vi "Begin.vi"() -> (0 "error out":errorcluster)   [LabVIEW 2011]
doc: "Called before other user functions, this VI is expected to open initial I/O refnums, load in file data, and do all program initialization. Notice that the <B>error out</B> terminal is simply used for data flow. Wiring it to other structures or subVIs ensures that this VI runs first."
uses:
  <vilib>/Rock Robotics/WPI/Camera/WPI_CameraImageSize.ctl
  <vilib>/Rock Robotics/WPI/MotorControl/WPI_MotorControlDeviceRef.ctl
  <vilib>/Rock Robotics/SystemInterfaces/Typedef/FPGA_TypedefDigitalModule.ctl
  <vilib>/Rock Robotics/SystemInterfaces/DIO/FPGA_DIOPWMChannel.ctl
  <vilib>/Rock Robotics/WPI/PWM/WPI_PWMDeadband.ctl
  <vilib>/Rock Robotics/WPI/CAN/Jaguar/SubVIs/WPI_CANJaguar_ControlMode.ctl
  <vilib>/Rock Robotics/WPI/PWM/WPI_PWMTransform_ConPane.ctl
  PIDCluster.ctl
  <vilib>/Rock Robotics/SystemInterfaces/DIO/FPGA_DIORelayChannel.ctl
  <vilib>/Rock Robotics/WPI/Solenoid/WPI_SolenoidChannel.ctl
  <vilib>/Rock Robotics/SystemInterfaces/DIO/FPGA_DIOChannel.ctl
  <vilib>/Rock Robotics/WPI/Camera/WPI_CameraFrameRate.ctl
  <vilib>/Rock Robotics/WPI/Camera/WPI_CameraExposure Values.ctl
  <vilib>/Rock Robotics/WPI/Camera/WPI_CameraWhite Balance Values.ctl
  <vilib>/Rock Robotics/SystemInterfaces/AI/FPGA_AIGyroChannel.ctl
  <vilib>/Rock Robotics/SystemInterfaces/Typedef/FPGA_TypedefAnalogModule.ctl
  <vilib>/Rock Robotics/WPI/Joystick/WPI_JoystickDeviceEnum.ctl
  <vilib>/Rock Robotics/SystemInterfaces/Typedef/FPGA_TypedefSolenoidModule.ctl
  <vilib>/Rock Robotics/WPI/Solenoid/WPI_SolenoidOpenSingle.vi
  <vilib>/Rock Robotics/WPI/Counter/WPI_CounterDigitalInputToDigitalSource.vi
  <vilib>/Rock Robotics/WPI/Counter/WPI_CounterOpen UpDown Mode.vi
  <vilib>/Rock Robotics/WPI/MotorControl/WPI_MotorControlOpen Victor.vi
  <vilib>/Rock Robotics/WPI/MotorControl/WPI_MotorControlOpen Jaguar.vi
  <vilib>/Rock Robotics/WPI/Compressor/WPI_CompressorGetSetRefNum.vi
  <vilib>/Rock Robotics/WPI/Relay/WPI_RelayValue.ctl
  <vilib>/Rock Robotics/WPI/Relay/WPI_RelayDirection.ctl
panel:
  out "MotorControlDeviceRef":T1={"DeviceStatus"={"status"=FALSE, "code"=0, "source"=""}, "Type"=enum."PWM", "PWM"={"Digital Module"=enum."Digital Module 1", "PWM Channel"=enum."Invalid", "DeadBand"={"Name"="", "maxPositivePwm"=0, "minPositivePwm"=0, "centerPwm"=0, "maxNegativePwm"=0, "minNegativePwm"=0, "angularRange"=0}}, "CAN"={"Device Number"=0, "Control Mode"=enum."Percent VBus", "Semaphore"=refnum, "Max Vout"=12.0}, "Invert"=FALSE, "TransformRef"=refnum, "InvTransformRef"=refnum}
  in  "Image Size":T8=enum."320x240"
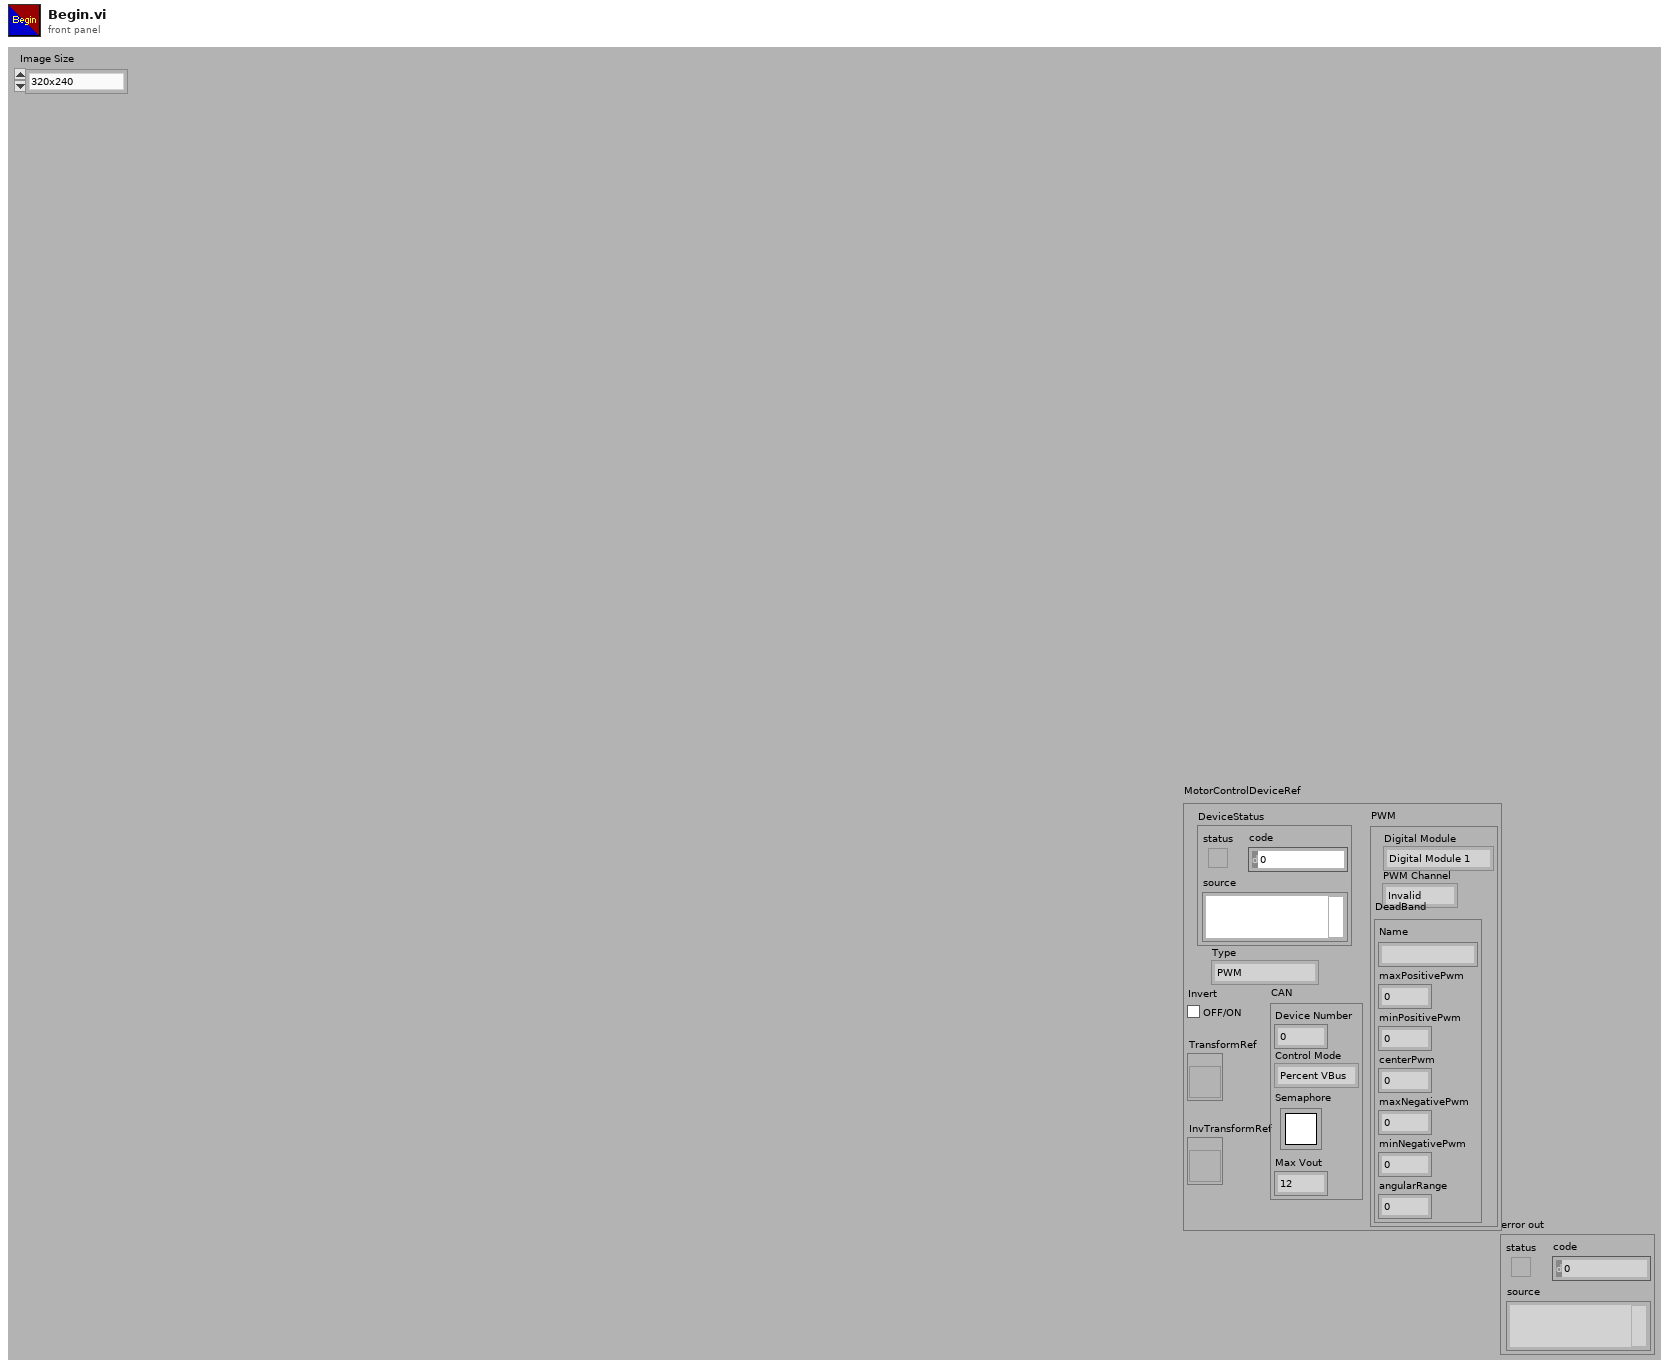
[diagram p1: front panel]
types:
  T1 = typedef "WPI_MotorControlDeviceRef.ctl" = cluster{"DeviceStatus":errorcluster, "Type":enum16{"PWM", "CAN"}, "PWM":cluster{"Digital Module":T2, "PWM Channel":T3, "DeadBand":T4}, "CAN":cluster{"Device Number":u8, "Control Mode":T5, "Semaphore":T6, "Max Vout":dbl}, "Invert":bool, "TransformRef":T7, "InvTransformRef":T7}
  T2 = typedef "FPGA_TypedefDigitalModule.ctl" = enum16{"Digital Module 1", "Digital Module 2"}
  T3 = typedef "FPGA_DIOPWMChannel.ctl" = enum8{"PWM 1", "PWM 2", "PWM 3", "PWM 4", "PWM 5", "PWM 6", "PWM 7", "PWM 8", "PWM 9", "PWM 10", "Invalid"}
  T4 = typedef "WPI_PWMDeadband.ctl" = cluster{"Name":string, "maxPositivePwm":i32, "minPositivePwm":i32, "centerPwm":i32, "maxNegativePwm":i32, "minNegativePwm":i32, "angularRange":u16}
  T5 = typedef "WPI_CANJaguar_ControlMode.ctl" = enum8{"Percent VBus", "Current", "Speed", "Position", "Voltage"}
  T6 = typedef "Semaphore RefNum" = refnum<k1>
  T7 = typedef "WPI_PWMTransform_ConPane.ctl" = refnum<vi>
  T8 = typedef "WPI_CameraImageSize.ctl" = enum16{"640x480", "320x240", "160x120"}
  T9 = typedef "PIDCluster.ctl" = cluster{"P":dbl, "I":dbl, "D":dbl}
  T10 = typedef "FPGA_DIORelayChannel.ctl" = enum8{"Relay 1", "Relay 2", "Relay 3", "Relay 4", "Relay 5", "Relay 6", "Relay 7", "Relay 8", "Invalid"}
  T11 = typedef "WPI_SolenoidChannel.ctl" = enum8{"Solenoid 1", "Solenoid 2", "Solenoid 3", "Solenoid 4", "Solenoid 5", "Solenoid 6", "Solenoid 7", "Solenoid 8", "Invalid"}
  T12 = typedef "FPGA_TypedefSolenoidModule.ctl" = enum16{"Solenoid Module 1", "Solenoid Module 2"}
  T13 = typedef "FPGA_DIOChannel.ctl" = enum8{"DIO 1", "DIO 2", "DIO 3", "DIO 4", "DIO 5", "DIO 6", "DIO 7", "DIO 8", "DIO 9", "DIO 10", "DIO 11", "DIO 12", "DIO 13", "DIO 14", "Invalid"}
  T14 = typedef "WPI_CameraFrameRate.ctl" = u32
  T15 = typedef "WPI_CameraExposure Values.ctl" = enum16{"Auto", "Flicker-free 50 Hz", "Flicker-free 60 Hz", "Hold current"}
  T16 = typedef "WPI_CameraWhite Balance Values.ctl" = enum16{"Auto", "Fixed indoor", "Fixed outdoor 1", "Fixed outdoor 2", "Fixed fluorescent 1", "Fixed fluorescent 2", "Hold current"}
  T17 = typedef "FPGA_AIGyroChannel.ctl" = enum8{"AI 1", "AI 2", "Invalid"}
  T18 = typedef "FPGA_TypedefAnalogModule.ctl" = enum16{"Analog Module 1", "Analog Module 2"}
  T19 = typedef "WPI_JoystickDeviceEnum.ctl" = enum16{"USB 1", "USB 2", "USB 3", "USB 4", "Kinect 1", "Kinect 2"}
  T20 = typedef "WPI_RelayDirection.ctl" = enum16{"Both directions", "Forward only", "Reverse only"}
  T21 = typedef "WPI_RelayValue.ctl" = enum16{"Off", "On", "Forward", "Reverse"}
  T22 = typedef "WPI_I2CDevRef.ctl" = cluster{"DevStatus":errorcluster, "Digital Module":T2, "Device Address":u8}
  T23 = typedef "WPI_DigitalInputDevRef.ctl" = cluster{"DevStatus":errorcluster, "DIO Channel":T13, "Digital Module":T2}
  T24 = typedef "FPGA_CounterEncoderSourceConvertionLVSourceType.ctl" = cluster{"DevStatus":errorcluster, "AnalogTriggerMode?":bool, "DigitalMode":cluster{"Digital Module":T2, "DIO Channel":T25}, "AnalogTriggerMode":cluster{"AnalogTriggerIndex":T26, "OutputType":T27}}
  T25 = typedef "FPGA_DIODigitalSourceChannel.ctl" = enum8{"DIO 1", "DIO 2", "DIO 3", "DIO 4", "DIO 5", "DIO 6", "DIO 7", "DIO 8", "DIO 9", "DIO 10", "DIO 11", "DIO 12", "DIO 13", "DIO 14", "Disabled"}
  T26 = typedef "FPGA_AnalogTriggerIndex.ctl" = enum8{"Trig 0", "Trig 1", "Trig 2", "Trig 3", "Trig 4", "Trig 5", "Trig 6", "Trig 7", "Invalid"}
  T27 = typedef "FPGA_AnalogTriggerOutType.ctl" = enum16{"InWindow", "TriggerState", "Rising", "Falling"}
  T28 = typedef "WPI_SolenoidDevRef.ctl" = cluster{"DevStatus":errorcluster, "Solenoid Module":T12, "Forward Solenoid Channel":T11, "Reverse Solenoid Channel":T11}
  T29 = typedef "WPI_CounterDevRef.ctl" = cluster{"DevStatus":errorcluster, "CntIndex":T30}
  T30 = typedef "FPGA_CounterCtrSystemIndex.ctl" = enum8{"Ctr 0", "Ctr 1", "Ctr 2", "Ctr 3", "Ctr 4", "Ctr 5", "Ctr 6", "Ctr 7", "Invalid"}
  T31 = typedef "WPI_GyroDevRef.ctl" = cluster{"DevStatus":errorcluster, "Analog Module":T18, "Analog Channel":T32, "Offset":dbl, "Gain (VoltsPerDegree/Second)":dbl}
  T32 = typedef "FPGA_AIChannel.ctl" = enum8{"AI 1", "AI 2", "AI 3", "AI 4", "AI 5", "AI 6", "AI 7", "AI 8", "Invalid"}
  T33 = typedef "WPI_CompressorDevRef.ctl" = cluster{"DevStatus":errorcluster, "DigitalInputDevRef":T23, "RelayDevRef":T34}
  T34 = typedef "WPI_RelayDevRef.ctl" = cluster{"DevStatus":errorcluster, "Relay Channel":T10, "Digital Module":T2, "Relay Direction":T20}
  T35 = typedef "WPI_DigitalOutputDevRef.ctl" = cluster{"Digital Module":T2, "DIO Channel":T13, "DevStatus":errorcluster}
  T36 = typedef "WPI_CameraDevRef.ctl" = cluster{"Camera Address":string, "CameraStatus":errorcluster, "Acquire Image Notifier":refnum<notifier>}
  T37 = typedef "WPI_JoystickDevRef.ctl" = cluster{"Device":T19}
  T38 = typedef "WPI_EncoderDevRef.ctl" = cluster{"DevStatus":errorcluster, "EncoderIndex":T39, "CounterIndex":T30, "DistancePerCount":dbl, "Decoding Type":T40}
  T39 = typedef "FPGA_EncoderIdx.ctl" = enum8{"Enc 0", "Enc 1", "Enc 2", "Enc 3", "Invalid"}
  T40 = typedef "WPI_EncoderType.ctl" = enum16{"1x", "2x", "4x"}
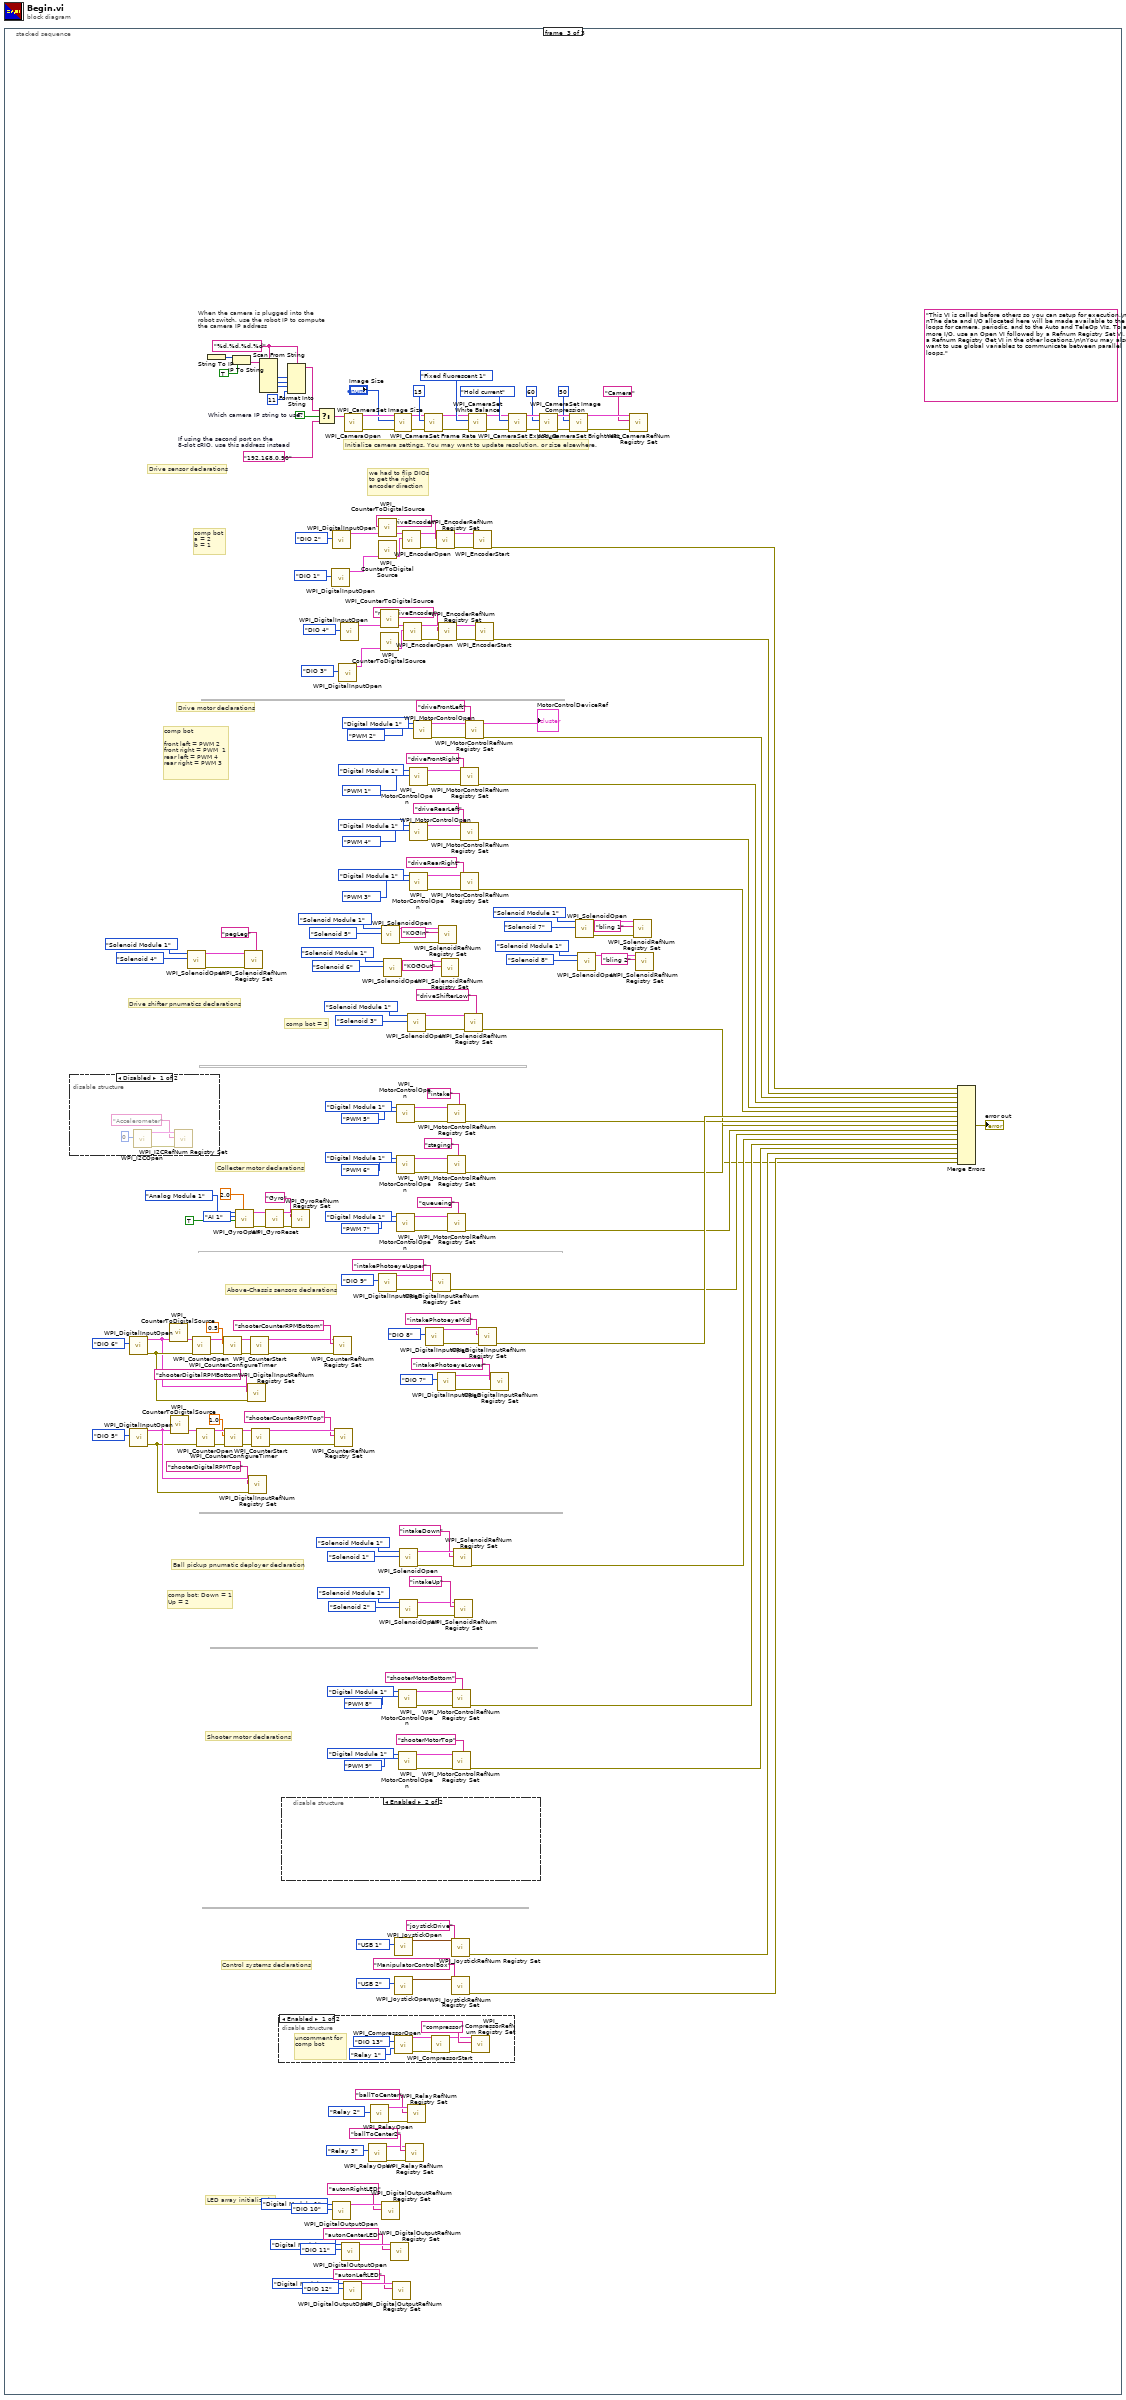
[diagram p0: block diagram]
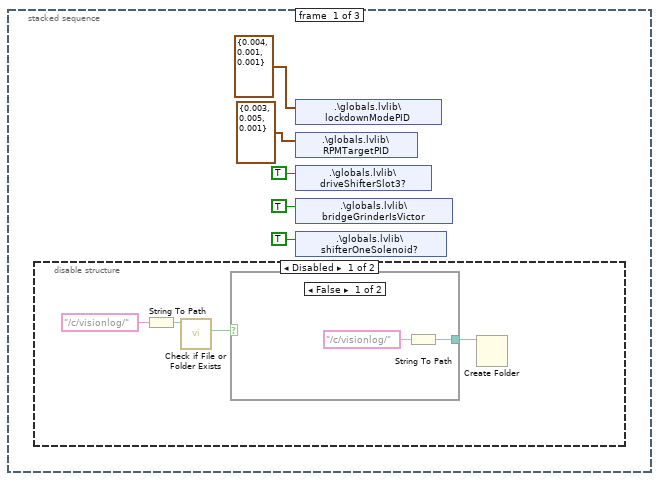
[diagram p2: hidden frame]
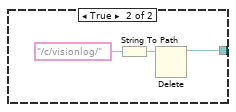
[diagram p3: hidden frame]
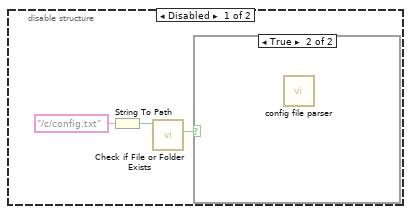
[diagram p6: hidden frame]
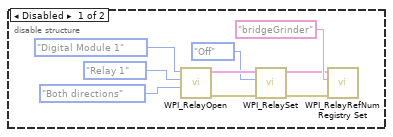
[diagram p10: hidden frame]
diagram:
  n1 = stacked-sequence {
    frame #0 {
      n2 = disable-structure shown="Disabled" {
        frame Disabled {
          n3 = String To Path(string="/c/visionlog/") -> (path=w8:path)
          n4 = call <vilib>:"Check if File or Folder Exists.vi"("path"=w8) -> ("file or folder exists?"=w7:bool)  [unwired: 8 in, 2 out]
          n5 = case shown="False" w7 {
            tunnel: [w10 w12] -> w6
            frame False {
              n6 = String To Path(string="/c/visionlog/") -> (path=w10:path)
            }
            frame True {
              n7 = String To Path(string="/c/visionlog/") -> (path=w13:path)
              n8 = Delete(path (use dialog)=w13) -> (deleted path=w12:path)  [unwired: 4 in, 2 out]
            }
          }
          n9 = Create Folder(path (use dialog)=w6) -> ()  [unwired: 2 in, 3 out]
        }
        frame Enabled {
        }
      }
      n10 = shared-variable ".\\globals.lvlib\\lockdownModePID"(T9 {"P"=0.004, "I"=0.001, "D"=0.001} ("lockdownModePID")) -> ()  [unwired: 1 in, 1 out]
      n11 = shared-variable ".\\globals.lvlib\\RPMTargetPID"(T9 {"P"=0.003, "I"=0.005, "D"=0.001} ("RPMTargetPID")) -> ()  [unwired: 1 in, 1 out]
      n12 = shared-variable ".\\globals.lvlib\\driveShifterSlot3?"(TRUE ("driveShifterSlot3?")) -> ()  [unwired: 1 in, 1 out]
      n13 = shared-variable ".\\globals.lvlib\\bridgeGrinderIsVictor"(TRUE ("bridgeGrinderIsVictor")) -> ()  [unwired: 1 in, 1 out]
      n14 = shared-variable ".\\globals.lvlib\\shifterOneSolenoid?"(TRUE ("shifterOneSolenoid?")) -> ()  [unwired: 1 in, 1 out]
    }
    frame #1 {
      n15 = disable-structure shown="Enabled" {
        frame Disabled {
          n16 = String To Path(string="/c/config.txt") -> (path=w16:path)
          n17 = call <vilib>:"Check if File or Folder Exists.vi"("path"=w16) -> ("file or folder exists?"=w15:bool)  [unwired: 8 in, 2 out]
          n18 = case shown="True" w15 {
            frame False {
            }
            frame True {
              n19 = call "config file parser.vi"() -> ()  [unwired: 12 in]
            }
          }
        }
        frame Enabled {
        }
      }
    }
    frame #2 {
      w223 = TRUE  # Which camera IP string to use?
      w219 = "%d.%d.%d.%d" ("format string")
      w222 = "192.168.0.90"  # If using the second port on the 8-slot cRIO, use this address instead
      (unwired) "This VI is called before others so you can setup for execution.\n\nThe data and I/O allocated here will be made available to the loops for camera, periodic, and to the Auto and TeleOp VIs. To add more I/O, use an Open VI followed by a Refnum Registry Set VI.  Use a Refnum Registry Get VI in the other locations.\n\nYou may also want to use global variables to communicate between parallel loops."
      # "comp bot\na = 2\nb = 1"
      # "comp bot = 3"
      # "comp bot: Down = 1\nUp = 2"
      # "LED array initialization"
      # "comp bot\n\nfront left = PWM 2\nfront right = PWM  1\nrear left = PWM 4\nrear right = PWM 3"
      # "When the camera is plugged into the\nrobot switch, use the robot IP to compute\nthe camera IP address"
      # "Initialize camera settings. You may want to update resolution, or size elsewhere."
      # "we had to flip DIOs to get the right encoder direction"
      # "Control systems declarations"
      # "Drive sensor declarations"
      # "Shooter motor declarations"
      # "Ball pickup pnumatic deployer declaration"
      # "Above-Chassis sensors declarations"
      # "Collecter motor declarations"
      # "Drive shifter pnumatics declarations"
      # "Drive motor declarations"
      n20 = disable-structure shown="Disabled" {
        frame Disabled {
          n21 = call <vilib>:"WPI_I2COpen.vi"("Device Address"=u8 0) -> ("error out"=w255:errorcluster, "I2CDevRef"=w256:T22)  [unwired: 9 in]
          n22 = call <vilib>:"WPI_I2CRefNum Registry Set.vi"("error in (no error)"=w255, "refnum name"="Accelerometer", "I2CDevRef"=w256) -> ()  [unwired: 7 in, 2 out]
        }
        frame Enabled {
        }
      }
      n23 = call <vilib>:"WPI_DigitalInputOpen.vi"("DIO Channel"=FPGA_DIOChannel."DIO 6") -> ("error out"=w149:errorcluster, "DigitalInputDevRef"=w146:T23)  [unwired: 9 in]
      n24 = call <vilib>:"WPI_DigitalInputOpen.vi"("DIO Channel"=FPGA_DIOChannel."DIO 5") -> ("error out"=w166:errorcluster, "DigitalInputDevRef"=w169:T23)  [unwired: 9 in]
      n25 = call-poly <vilib>:"WPI_CounterToDigitalSource.vi"("DigitalInputDevRef"=w146) -> ("Digital Source"=w148:T24)  [unwired: 6 in]
      n26 = call-poly <vilib>:"WPI_CounterToDigitalSource.vi"("DigitalInputDevRef"=w169) -> ("Digital Source"=w167:T24)  [unwired: 6 in]
      n27 = call-poly <vilib>:"WPI_SolenoidOpen.vi"("Solenoid Channel"=WPI_SolenoidChannel."Solenoid 4" ("Forward Solenoid Channel"), "Solenoid Module (Module 1)"=FPGA_TypedefSolenoidModule."Solenoid Module 1") -> ("error out"=w35:errorcluster, "SolenoidDevRef"=w36:T28)  [unwired: 8 in]
      n28 = call-poly <vilib>:"WPI_CounterOpen.vi"("error in (no error)"=w149, "Up Source"=w148) -> ("error out"=w151:errorcluster, "CounterDevRef"=w150:T29)  [unwired: 8 in]
      n29 = call-poly <vilib>:"WPI_CounterOpen.vi"("error in (no error)"=w166, "Up Source"=w167) -> ("error out"=w164:errorcluster, "CounterDevRef"=w165:T29)  [unwired: 8 in]
      n30 = String To IP() -> (0:w212:u32)  [unwired: 1 in]
      n31 = call <vilib>:"WPI_CounterConfigureTimer.vi"("error in (no error)"=w151, "MaxPeriod (sec)"=0.5, "CounterDevRef in"=w150) -> ("error out"=w153:errorcluster, "CounterDevRef out"=w154:T29)  [unwired: 7 in]
      n32 = call <vilib>:"WPI_CounterConfigureTimer.vi"("error in (no error)"=w164, "MaxPeriod (sec)"=1.0, "CounterDevRef in"=w165) -> ("error out"=w162:errorcluster, "CounterDevRef out"=w161:T29)  [unwired: 7 in]
      n33 = IP To String(1:TRUE ("dot notation? (F)"), 2:w212) -> (0:w214:string)
      n34 = call <vilib>:"WPI_GyroOpen.vi"("Calibration Time (s)"=2.0, "Calibrate On Open"=TRUE, "Analog Channel"=FPGA_AIGyroChannel."AI 1", "Analog Module (Module 1)"=FPGA_TypedefAnalogModule."Analog Module 1") -> ("error out"=w181:errorcluster, "GyroDevRef"=w178:T31)  [unwired: 5 in, 1 out]
      n35 = call <vilib>:"WPI_SolenoidRefNum Registry Set.vi"("error in (no error)"=w35, "refnum name"="pegLeg", "SolenoidDevRef"=w36) -> ()  [unwired: 7 in, 2 out]
      n36 = call <vilib>:"WPI_DigitalInputRefNum Registry Set.vi"("error in (no error)"=w149, "refnum name"="shooterDigitalRPMBottom", "DigitalInputDevRef"=w146) -> ()  [unwired: 7 in, 2 out]
      n37 = call <vilib>:"WPI_DigitalInputRefNum Registry Set.vi"("error in (no error)"=w166, "refnum name"="shooterDigitalRPMTop", "DigitalInputDevRef"=w169) -> ()  [unwired: 7 in, 2 out]
      n38 = call <vilib>:"WPI_CounterStart.vi"("error in (no error)"=w153, "CounterDevRef in"=w154) -> ("error out"=w156:errorcluster, "CounterDevRef out"=w155:T29)  [unwired: 8 in]
      n39 = call <vilib>:"WPI_CounterStart.vi"("error in (no error)"=w162, "CounterDevRef in"=w161) -> ("error out"=w159:errorcluster, "CounterDevRef out"=w160:T29)  [unwired: 8 in]
      n40 = Scan From String(format string=w219, input string=w214) -> (output 1=w215:i32, output 2=w216:i32, output 3=w217:i32)  [unwired: 7 in, 3 out]
      n41 = call <vilib>:"WPI_GyroReset.vi"("error in (no error)"=w181, "GyroDevRef"=w178) -> ("error out"=w180:errorcluster, "GyroDevRef"=w179:T31)  [unwired: 8 in]
      n42 = disable-structure shown="Enabled" {
        frame Enabled {
          # "uncomment for comp bot"
          n43 = call <vilib>:"WPI_CompressorOpen.vi"("Pressure Switch DIO Channel"=FPGA_DIOChannel."DIO 13", "Relay Channel"=FPGA_DIORelayChannel."Relay 1") -> ("CompressorDevRef"=w250:T33, "error out"=w247:errorcluster)  [unwired: 12 in]
          n44 = call <vilib>:"WPI_CompressorStart.vi"("error in (no error)"=w247, "CompressorDevRef"=w250) -> ("error out"=w248:errorcluster, "CompressorDevRef"=w249:T33)  [unwired: 8 in]
          n45 = call <vilib>:"WPI_CompressorRefNum Registry Set.vi"("error in (no error)"=w248, "refnum name"="compressor", "CompressorDevRef"=w249) -> ()  [unwired: 7 in, 2 out]
        }
        frame Disabled {
        }
      }
      n46 = disable-structure shown="Enabled" {
        frame Disabled {
          n47 = call <vilib>:"WPI_RelayOpen.vi"("Relay Direction"=WPI_RelayDirection."Both directions", "Relay Channel"=FPGA_DIORelayChannel."Relay 1", "Digital Module (Module 1)"=FPGA_TypedefDigitalModule."Digital Module 1") -> ("error out"=w263:errorcluster, "RelayDevRef"=w262:T34)  [unwired: 7 in]
          n48 = call <vilib>:"WPI_RelaySet.vi"("error in (no error)"=w263, "RelayValue"=WPI_RelayValue."Off", "RelayDevRef"=w262) -> ("error out"=w265:errorcluster, "RelayDevRef"=w264:T34)  [unwired: 7 in]
          n49 = call <vilib>:"WPI_RelayRefNum Registry Set.vi"("error in (no error)"=w265, "refnum name"="bridgeGrinder", "RelayDevRef"=w264) -> ()  [unwired: 7 in, 2 out]
        }
        frame Enabled {
        }
      }
      n50 = Format Into String(format string=w219, w215, w216, w217, 11 ("Compression")) -> (resulting string=w221:string)  [unwired: 2 in, 1 out]
      n51 = call <vilib>:"WPI_GyroRefNum Registry Set.vi"("error in (no error)"=w180, "refnum name"="Gyro", "GyroDevRef"=w179) -> ()  [unwired: 7 in, 2 out]
      n52 = Select(t=w221, s=w223, f=w222) -> (s? t:f=w220:string)
      n53 = call <vilib>:"WPI_DigitalInputOpen.vi"("DIO Channel"=FPGA_DIOChannel."DIO 1") -> ("DigitalInputDevRef"=w42:T23)  [unwired: 9 in, 1 out]
      n54 = call <vilib>:"WPI_DigitalInputOpen.vi"("DIO Channel"=FPGA_DIOChannel."DIO 2") -> ("DigitalInputDevRef"=w43:T23)  [unwired: 9 in, 1 out]
      n55 = call <vilib>:"WPI_DigitalOutputOpen.vi"("DIO Channel"=FPGA_DIOChannel."DIO 10", "Digital Module (Module 1)"=FPGA_TypedefDigitalModule."Digital Module 1") -> ("DigitalOutputDevRef"=w87:T35)  [unwired: 8 in, 1 out]
      n56 = call <vilib>:"WPI_CounterRefNum Registry Set.vi"("error in (no error)"=w156, "refnum name"="shooterCounterRPMBottom", "CounterDevRef"=w155) -> ()  [unwired: 7 in, 2 out]
      n57 = call <vilib>:"WPI_CounterRefNum Registry Set.vi"("error in (no error)"=w159, "refnum name"="shooterCounterRPMTop", "CounterDevRef"=w160) -> ()  [unwired: 7 in, 2 out]
      n58 = call <vilib>:"WPI_DigitalInputOpen.vi"("DIO Channel"=FPGA_DIOChannel."DIO 3") -> ("DigitalInputDevRef"=w40:T23)  [unwired: 9 in, 1 out]
      n59 = call <vilib>:"WPI_DigitalInputOpen.vi"("DIO Channel"=FPGA_DIOChannel."DIO 4") -> ("DigitalInputDevRef"=w41:T23)  [unwired: 9 in, 1 out]
      n60 = call <vilib>:"WPI_DigitalOutputOpen.vi"("DIO Channel"=FPGA_DIOChannel."DIO 11", "Digital Module (Module 1)"=FPGA_TypedefDigitalModule."Digital Module 1") -> ("DigitalOutputDevRef"=w84:T35)  [unwired: 8 in, 1 out]
      n61 = call <vilib>:"WPI_DigitalOutputOpen.vi"("DIO Channel"=FPGA_DIOChannel."DIO 12", "Digital Module (Module 1)"=FPGA_TypedefDigitalModule."Digital Module 1") -> ("DigitalOutputDevRef"=w83:T35)  [unwired: 8 in, 1 out]
      n62 = call <vilib>:"WPI_CameraOpen.vi"("Camera Address"=w220) -> ("error out"=w201:errorcluster, "CameraDevRef"=w200:T36)  [unwired: 1 in, 8 out]
      n63 = call <vilib>:"WPI_RelayOpen.vi"("Relay Channel"=FPGA_DIORelayChannel."Relay 3") -> ("error out"=w19:errorcluster, "RelayDevRef"=w18:T34)  [unwired: 9 in]
      n64 = call <vilib>:"WPI_RelayOpen.vi"("Relay Channel"=FPGA_DIORelayChannel."Relay 2") -> ("error out"=w33:errorcluster, "RelayDevRef"=w34:T34)  [unwired: 9 in]
      n65 = call-poly <vilib>:"WPI_CounterToDigitalSource.vi"("DigitalInputDevRef"=w43) -> ("Digital Source"=w72:T24)  [unwired: 6 in]
      n66 = call-poly <vilib>:"WPI_CounterToDigitalSource.vi"("DigitalInputDevRef"=w42) -> ("Digital Source"=w73:T24)  [unwired: 6 in]
      n67 = call <vilib>:"WPI_DigitalInputOpen.vi"("DIO Channel"=FPGA_DIOChannel."DIO 9") -> ("error out"=w191:errorcluster, "DigitalInputDevRef"=w143:T23)  [unwired: 9 in]
      n68 = call-poly <vilib>:"WPI_CounterToDigitalSource.vi"("DigitalInputDevRef"=w41) -> ("Digital Source"=w75:T24)  [unwired: 6 in]
      n69 = call-poly <vilib>:"WPI_CounterToDigitalSource.vi"("DigitalInputDevRef"=w40) -> ("Digital Source"=w74:T24)  [unwired: 6 in]
      n70 = call-poly <vilib>:"WPI_SolenoidOpen.vi"("Solenoid Channel"=WPI_SolenoidChannel."Solenoid 5" ("Forward Solenoid Channel"), "Solenoid Module (Module 1)"=FPGA_TypedefSolenoidModule."Solenoid Module 1") -> ("error out"=w30:errorcluster, "SolenoidDevRef"=w29:T28)  [unwired: 8 in]
      n71 = call <vilib>:"WPI_DigitalOutputRefNum Registry Set.vi"("refnum name"="autonRightLED", "DigitalOutputDevRef"=w87) -> ()  [unwired: 8 in, 2 out]
      n72 = call-poly <vilib>:"WPI_SolenoidOpen.vi"("Solenoid Channel"=WPI_SolenoidChannel."Solenoid 6" ("Forward Solenoid Channel"), "Solenoid Module (Module 1)"=FPGA_TypedefSolenoidModule."Solenoid Module 1") -> ("SolenoidDevRef"=w22:T28)  [unwired: 8 in, 1 out]
      n73 = call <vilib>:"WPI_DigitalOutputRefNum Registry Set.vi"("refnum name"="autonCenterLED", "DigitalOutputDevRef"=w84) -> ()  [unwired: 8 in, 2 out]
      n74 = call <vilib>:"WPI_DigitalOutputRefNum Registry Set.vi"("refnum name"="autonLeftLED", "DigitalOutputDevRef"=w83) -> ()  [unwired: 8 in, 2 out]
      n75 = call <vilib>:"WPI_CameraSet Image Size.vi"("error in (no error)"=w201, "Image Size"="Image Size", "CameraDevRef"=w200) -> ("error out"=w202:errorcluster, "CameraDevRef Out"=w199:T36)  [unwired: 7 out]
      n76 = call <vilib>:"WPI_JoystickOpen.vi"("JoystickDevice"=WPI_JoystickDeviceEnum."USB 1") -> ("JoystickDevRef"=w88:T37)  [unwired: 10 in]
      n77 = call <vilib>:"WPI_JoystickOpen.vi"("JoystickDevice"=WPI_JoystickDeviceEnum."USB 2") -> ("JoystickDevRef"=w135:T37)  [unwired: 10 in]
      n78 = call-poly <vilib>:"WPI_MotorControlOpen.vi"("PWM Channel"=FPGA_DIOPWMChannel."PWM 5", "Digital Module (Module 1)"=FPGA_TypedefDigitalModule."Digital Module 1") -> ("error out"=w188:errorcluster, "MotorControlDeviceRef"=w95:T1)  [unwired: 8 in]
      n79 = call-poly <vilib>:"WPI_MotorControlOpen.vi"("PWM Channel"=FPGA_DIOPWMChannel."PWM 6", "Digital Module (Module 1)"=FPGA_TypedefDigitalModule."Digital Module 1") -> ("error out"=w189:errorcluster, "MotorControlDeviceRef"=w99:T1)  [unwired: 8 in]
      n80 = call-poly <vilib>:"WPI_MotorControlOpen.vi"("PWM Channel"=FPGA_DIOPWMChannel."PWM 7", "Digital Module (Module 1)"=FPGA_TypedefDigitalModule."Digital Module 1") -> ("error out"=w190:errorcluster, "MotorControlDeviceRef"=w134:T1)  [unwired: 8 in]
      n81 = call-poly <vilib>:"WPI_MotorControlOpen.vi"("PWM Channel"=FPGA_DIOPWMChannel."PWM 8", "Digital Module (Module 1)"=FPGA_TypedefDigitalModule."Digital Module 1") -> ("error out"=w183:errorcluster, "MotorControlDeviceRef"=w114:T1)  [unwired: 8 in]
      n82 = call-poly <vilib>:"WPI_MotorControlOpen.vi"("PWM Channel"=FPGA_DIOPWMChannel."PWM 9", "Digital Module (Module 1)"=FPGA_TypedefDigitalModule."Digital Module 1") -> ("error out"=w246:errorcluster, "MotorControlDeviceRef"=w110:T1)  [unwired: 8 in]
      n83 = call-poly <vilib>:"WPI_SolenoidOpen.vi"("Solenoid Channel"=WPI_SolenoidChannel."Solenoid 1" ("Forward Solenoid Channel"), "Solenoid Module (Module 1)"=FPGA_TypedefSolenoidModule."Solenoid Module 1") -> ("error out"=w182:errorcluster, "SolenoidDevRef"=w106:T28)  [unwired: 8 in]
      n84 = call-poly <vilib>:"WPI_SolenoidOpen.vi"("Solenoid Channel"=WPI_SolenoidChannel."Solenoid 2" ("Forward Solenoid Channel"), "Solenoid Module (Module 1)"=FPGA_TypedefSolenoidModule."Solenoid Module 1") -> ("error out"=w232:errorcluster, "SolenoidDevRef"=w233:T28)  [unwired: 8 in]
      n85 = call <vilib>:"WPI_EncoderOpen.vi"("BSource"=w73, "ASource"=w72) -> ("error out"=w67:errorcluster, "EncoderDevRef"=w68:T38)  [unwired: 8 in]
      n86 = call <vilib>:"WPI_EncoderOpen.vi"("BSource"=w74, "ASource"=w75) -> ("error out"=w142:errorcluster, "EncoderDevRef"=w141:T38)  [unwired: 8 in]
      n87 = call <vilib>:"WPI_RelayRefNum Registry Set.vi"("error in (no error)"=w19, "refnum name"="ballToCenter2", "RelayDevRef"=w18) -> ()  [unwired: 7 in, 2 out]
      n88 = call-poly <vilib>:"WPI_SolenoidOpen.vi"("Solenoid Channel"=WPI_SolenoidChannel."Solenoid 3" ("Forward Solenoid Channel"), "Solenoid Module (Module 1)"=FPGA_TypedefSolenoidModule."Solenoid Module 1") -> ("error out"=w172:errorcluster, "SolenoidDevRef"=w94:T28)  [unwired: 8 in]
      n89 = call <vilib>:"WPI_RelayRefNum Registry Set.vi"("error in (no error)"=w33, "refnum name"="ballToCenter", "RelayDevRef"=w34) -> ()  [unwired: 7 in, 2 out]
      n90 = call-poly <vilib>:"WPI_MotorControlOpen.vi"("PWM Channel"=FPGA_DIOPWMChannel."PWM 1", "Digital Module (Module 1)"=FPGA_TypedefDigitalModule."Digital Module 1") -> ("error out"=w185:errorcluster, "MotorControlDeviceRef"=w116:T1)  [unwired: 8 in]
      n91 = call-poly <vilib>:"WPI_MotorControlOpen.vi"("PWM Channel"=FPGA_DIOPWMChannel."PWM 4", "Digital Module (Module 1)"=FPGA_TypedefDigitalModule."Digital Module 1") -> ("error out"=w186:errorcluster, "MotorControlDeviceRef"=w117:T1)  [unwired: 8 in]
      n92 = call-poly <vilib>:"WPI_MotorControlOpen.vi"("PWM Channel"=FPGA_DIOPWMChannel."PWM 3", "Digital Module (Module 1)"=FPGA_TypedefDigitalModule."Digital Module 1") -> ("error out"=w187:errorcluster, "MotorControlDeviceRef"=w115:T1)  [unwired: 8 in]
      n93 = call-poly <vilib>:"WPI_MotorControlOpen.vi"("PWM Channel"=FPGA_DIOPWMChannel."PWM 2", "Digital Module (Module 1)"=FPGA_TypedefDigitalModule."Digital Module 1") -> ("error out"=w184:errorcluster, "MotorControlDeviceRef"=w118:T1)  [unwired: 8 in]
      "MotorControlDeviceRef" <- w118
      n94 = call <vilib>:"WPI_CameraSet Frame Rate.vi"("error in (no error)"=w202, "Frame Rate (fps)"=T14 15, "CameraDevRef"=w199) -> ("error out"=w203:errorcluster, "CameraDevRef Out"=w197:T36)  [unwired: 7 out]
      n95 = call <vilib>:"WPI_DigitalInputOpen.vi"("DIO Channel"=FPGA_DIOChannel."DIO 8") -> ("error out"=w224:errorcluster, "DigitalInputDevRef"=w227:T23)  [unwired: 9 in]
      n96 = call <vilib>:"WPI_DigitalInputRefNum Registry Set.vi"("error in (no error)"=w191, "refnum name"="intakePhotoeyeUpper", "DigitalInputDevRef"=w143) -> ("error out"=w56:errorcluster)  [unwired: 7 in, 1 out]
      n97 = call <vilib>:"WPI_EncoderRefNum Registry Set.vi"("error in (no error)"=w67, "refnum name"="leftDriveEncoder", "EncoderDevRef"=w68) -> ("error out"=w70:errorcluster, "EncoderDevRef"=w71:T38)  [unwired: 7 in]
      n98 = call <vilib>:"WPI_DigitalInputOpen.vi"("DIO Channel"=FPGA_DIOChannel."DIO 7") -> ("error out"=w231:errorcluster, "DigitalInputDevRef"=w228:T23)  [unwired: 9 in]
      n99 = call <vilib>:"WPI_EncoderRefNum Registry Set.vi"("error in (no error)"=w142, "refnum name"="rightDriveEncoder", "EncoderDevRef"=w141) -> ("error out"=w139:errorcluster, "EncoderDevRef"=w138:T38)  [unwired: 7 in]
      n100 = call <vilib>:"WPI_SolenoidRefNum Registry Set.vi"("error in (no error)"=w30, "refnum name"="KOGIn", "SolenoidDevRef"=w29) -> ()  [unwired: 7 in, 2 out]
      n101 = call <vilib>:"WPI_SolenoidRefNum Registry Set.vi"("refnum name"="KOGOut", "SolenoidDevRef"=w22) -> ()  [unwired: 8 in, 2 out]
      n102 = call <vilib>:"WPI_MotorControlRefNum Registry Set.vi"("error in (no error)"=w188, "refnum name"="intake", "MotorControlDevRef"=w95) -> ("error out"=w59:errorcluster)  [unwired: 7 in, 1 out]
      n103 = call <vilib>:"WPI_MotorControlRefNum Registry Set.vi"("error in (no error)"=w189, "refnum name"="staging", "MotorControlDevRef"=w99) -> ("error out"=w58:errorcluster)  [unwired: 7 in, 1 out]
      n104 = call <vilib>:"WPI_MotorControlRefNum Registry Set.vi"("error in (no error)"=w190, "refnum name"="queueing", "MotorControlDevRef"=w134) -> ("error out"=w57:errorcluster)  [unwired: 7 in, 1 out]
      n105 = call <vilib>:"WPI_JoystickRefNum Registry Set.vi"("refnum name"="joystickDrive", "JoystickDevRef"=w88) -> ("error out"=w52:errorcluster)  [unwired: 8 in, 1 out]
      n106 = call <vilib>:"WPI_JoystickRefNum Registry Set.vi"("refnum name"="ManipulatorControlBox", "JoystickDevRef"=w135) -> ("error out"=w51:errorcluster)  [unwired: 8 in, 1 out]
      n107 = call <vilib>:"WPI_MotorControlRefNum Registry Set.vi"("error in (no error)"=w183, "refnum name"="shooterMotorBottom", "MotorControlDevRef"=w114) -> ("error out"=w54:errorcluster)  [unwired: 7 in, 1 out]
      n108 = call <vilib>:"WPI_MotorControlRefNum Registry Set.vi"("error in (no error)"=w246, "refnum name"="shooterMotorTop", "MotorControlDevRef"=w110) -> ("error out"=w53:errorcluster)  [unwired: 7 in, 1 out]
      n109 = call <vilib>:"WPI_SolenoidRefNum Registry Set.vi"("error in (no error)"=w182, "refnum name"="intakeDown", "SolenoidDevRef"=w106) -> ("error out"=w55:errorcluster)  [unwired: 7 in, 1 out]
      n110 = call <vilib>:"WPI_SolenoidRefNum Registry Set.vi"("error in (no error)"=w232, "refnum name"="intakeUp", "SolenoidDevRef"=w233) -> ()  [unwired: 7 in, 2 out]
      n111 = call <vilib>:"WPI_MotorControlRefNum Registry Set.vi"("error in (no error)"=w185, "refnum name"="driveFrontRight", "MotorControlDevRef"=w116) -> ("error out"=w62:errorcluster)  [unwired: 7 in, 1 out]
      n112 = call <vilib>:"WPI_MotorControlRefNum Registry Set.vi"("error in (no error)"=w186, "refnum name"="driveRearLeft", "MotorControlDevRef"=w117) -> ("error out"=w63:errorcluster)  [unwired: 7 in, 1 out]
      n113 = call <vilib>:"WPI_MotorControlRefNum Registry Set.vi"("error in (no error)"=w187, "refnum name"="driveRearRight", "MotorControlDevRef"=w115) -> ("error out"=w61:errorcluster)  [unwired: 7 in, 1 out]
      n114 = call <vilib>:"WPI_SolenoidRefNum Registry Set.vi"("error in (no error)"=w172, "refnum name"="driveShifterLow", "SolenoidDevRef"=w94) -> ("error out"=w50:errorcluster)  [unwired: 7 in, 1 out]
      n115 = call <vilib>:"WPI_MotorControlRefNum Registry Set.vi"("error in (no error)"=w184, "refnum name"="driveFrontLeft", "MotorControlDevRef"=w118) -> ("error out"=w64:errorcluster)  [unwired: 7 in, 1 out]
      n116 = call <vilib>:"WPI_CameraSet White Balance.vi"("error in (no error)"=w203, "White Balance"=WPI_CameraWhite_Balance_Values."Fixed fluorescent 1", "CameraDevRef"=w197) -> ("error out"=w204:errorcluster, "CameraDevRef Out"=w198:T36)  [unwired: 7 out]
      n117 = call <vilib>:"WPI_EncoderStart.vi"("error in (no error)"=w70, "EncoderDevRef"=w71) -> ("error out"=w66:errorcluster)  [unwired: 8 in, 1 out]
      n118 = call <vilib>:"WPI_EncoderStart.vi"("error in (no error)"=w139, "EncoderDevRef"=w138) -> ("error out"=w65:errorcluster)  [unwired: 8 in, 1 out]
      n119 = call <vilib>:"WPI_DigitalInputRefNum Registry Set.vi"("error in (no error)"=w224, "refnum name"="intakePhotoeyeMid", "DigitalInputDevRef"=w227) -> ("error out"=w60:errorcluster)  [unwired: 7 in, 1 out]
      n120 = call <vilib>:"WPI_DigitalInputRefNum Registry Set.vi"("error in (no error)"=w231, "refnum name"="intakePhotoeyeLower", "DigitalInputDevRef"=w228) -> ()  [unwired: 7 in, 2 out]
      n121 = call <vilib>:"WPI_CameraSet Exposure.vi"("error in (no error)"=w204, "Exposure"=WPI_CameraExposure_Values."Hold current", "CameraDevRef"=w198) -> ("error out"=w205:errorcluster, "CameraDevRef Out"=w195:T36)  [unwired: 7 out]
      n122 = call <vilib>:"WPI_CameraSet Image Compression.vi"("error in (no error)"=w205, "Compression"=60, "CameraDevRef"=w195) -> ("error out"=w206:errorcluster, "CameraDevRef Out"=w196:T36)  [unwired: 7 out]
      n123 = call <vilib>:"WPI_CameraSet Brightness.vi"("error in (no error)"=w206, "Brightness"=50, "CameraDevRef"=w196) -> ("error out"=w208:errorcluster, "CameraDevRef Out"=w207:T36)  [unwired: 7 out]
      n124 = call-poly <vilib>:"WPI_SolenoidOpen.vi"("Solenoid Channel"=WPI_SolenoidChannel."Solenoid 7" ("Forward Solenoid Channel"), "Solenoid Module (Module 1)"=FPGA_TypedefSolenoidModule."Solenoid Module 1") -> ("error out"=w237:errorcluster, "SolenoidDevRef"=w238:T28)  [unwired: 8 in]
      n125 = call-poly <vilib>:"WPI_SolenoidOpen.vi"("Solenoid Channel"=WPI_SolenoidChannel."Solenoid 8" ("Forward Solenoid Channel"), "Solenoid Module (Module 1)"=FPGA_TypedefSolenoidModule."Solenoid Module 1") -> ("SolenoidDevRef"=w245:T28)  [unwired: 8 in, 1 out]
      n126 = call <vilib>:"WPI_CameraRefNum Registry Set.vi"("error in (no error)"=w208, "refnum name"="Camera", "CameraDevRef"=w207) -> ()  [unwired: 9 out]
      n127 = call <vilib>:"WPI_SolenoidRefNum Registry Set.vi"("error in (no error)"=w237, "refnum name"="bling 1", "SolenoidDevRef"=w238) -> ()  [unwired: 7 in, 2 out]
      n128 = call <vilib>:"WPI_SolenoidRefNum Registry Set.vi"("refnum name"="bling 2", "SolenoidDevRef"=w245) -> ()  [unwired: 8 in, 2 out]
      n129 = Merge Errors(w66, w65, w64, w62, w63, w61, w60, w59, w58, w57, w56, w55, w54, w53, w52, w51, w50) -> (→"error out":errorcluster)
    }
  }
